vi "Send Request.vi"   [LabVIEW 2015, in "JSONRPC Server.lvclass"]
doc: "This sends a Request to the RPC Server.\n\nAsync does not wait for a response from the server.\n\nSync waits for a response from the server."
uses:
  JSONRPC Server.lvclass
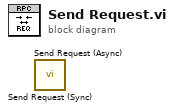
[diagram p0: block diagram]
diagram:
  n1 = call "Send Request (Sync).vi"() -> ()  [unwired: 9 in, 3 out]
  n2 = call "Send Request (Async).vi"() -> ()  [unwired: 8 in, 4 out]
